vi "DPO_7K_Max_and_Min_Vertical_Scale.vi"(10 "ATI?":bool) -> (0 "Min":dbl, 1 "Max":dbl)   [LabVIEW 2020]
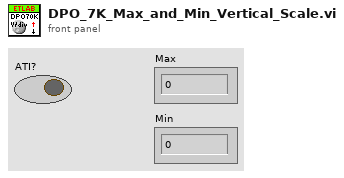
[diagram p1: front panel]
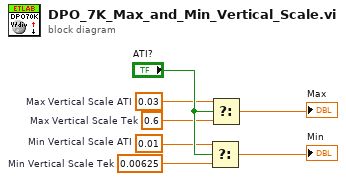
[diagram p0: block diagram]
diagram:
  w4 = 0.6  # Max Vertical Scale Tek
  w3 = 0.03  # Max Vertical Scale ATI
  w1 = 0.01  # Min Vertical Scale ATI
  w2 = 0.00625  # Min Vertical Scale Tek
  n1 = Select(t=w1, s="ATI?", f=w2) -> (s? t:f=→"Min":dbl)
  n2 = Select(t=w3, s="ATI?", f=w4) -> (s? t:f=→"Max":dbl)
